vi "left shift.vi"(11 "2048 2":dbl[][](array[numeric])) -> (3 "2048":dbl[][](array[numeric]))   [LabVIEW 2015]
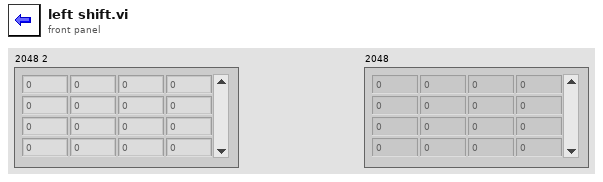
[diagram p1: front panel]
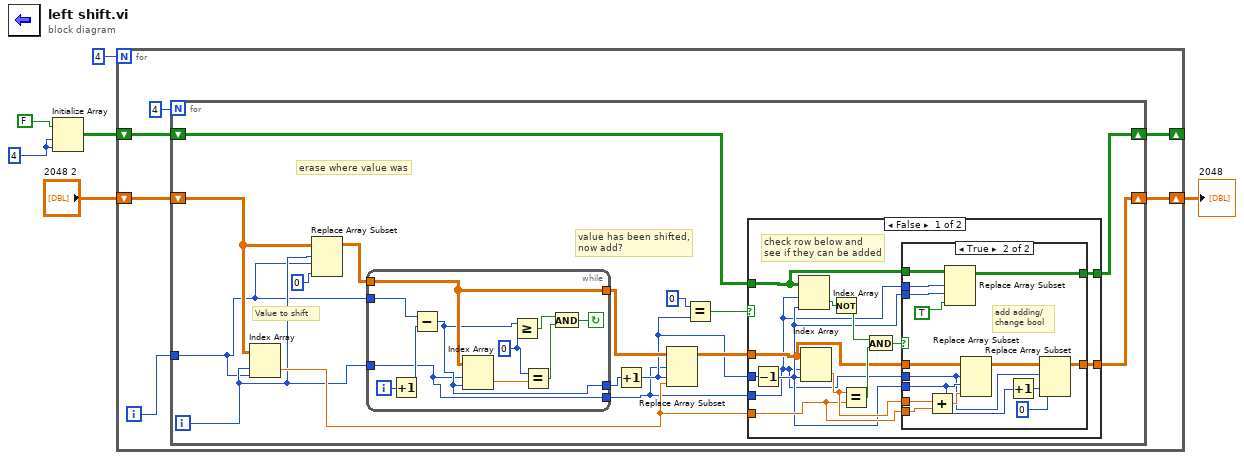
[diagram p0: block diagram]
diagram:
  w3 = 4
  n1 = Initialize Array(FALSE, w3, w3) -> (w1:bool[][])
  n2 = for {
    N: 4 -> [_]
    shift-right: [w8] -> _
    shift-left: w1 -> [w9]
    shift-right: [w7] -> w4
    shift-left: "2048 2" -> [w11]
    i -> [w10]
    n3 = for {
      N: 4 -> [_]
      tunnel: w10 -> [w13]
      shift-right: [w21] -> w8
      shift-left: w9 -> [w22]
      shift-right: [w20] -> w7
      shift-left: w11 -> [w18]
      i -> [w14]
      # "erase where value was"
      # "value has been shifted,\nnow add?"
      # "Value to shift"
      n4 = Index Array(array=w18, index (row)=w14, index (col)=w13) -> (element=w23:dbl)
      n5 = Replace Array Subset(array=w18, new element=0, index (row)=w14, index (col)=w13) -> (w19:dbl[][])
      n6 = while {
        tunnel: w13 -> [w71]
        tunnel: w14 -> [w62]
        tunnel: w19 -> [w64]
        tunnel: [w62] -> w15
        tunnel: [w63] -> w24
        tunnel: [w64] -> w28
        i -> [w70]
        stop <- w66 continue-if-true
        w61 = 0
        n7 = Increment(x=w70) -> (x+1=w67:i32)
        n8 = Subtract(x=w71, y=w67) -> (x-y=w63:i32)
        n9 = Index Array(array=w64, index (row)=w62, index (col)=w63) -> (element=w69:dbl)
        n10 = Greater Or Equal?(x=w63, y=w61) -> (x >= y?=w65:bool)
        n11 = Equal?(x=w61, y=w69) -> (x = y?=w68:bool)
        n12 = And(x=w65, y=w68) -> (x .and. y?=w66:bool)
      }
      n13 = Increment(x=w24) -> (x+1=w16:i32)
      n14 = Replace Array Subset(array=w28, new element=w23, index (row)=w15, index (col)=w16) -> (w25:dbl[][])
      n15 = Equal?(x=0, y=w16) -> (x = y?=w26:bool)
      n16 = case shown="False" w26 {
        tunnel: w25 -> [w35 w59]
        tunnel: w15 -> [w29 _]
        tunnel: w16 -> [w41 _]
        tunnel: w23 -> [w33 _]
        tunnel: w22 -> [w37 w60]
        tunnel: [w32 w60] -> w21
        tunnel: [w31 w59] -> w20
        frame False {
          # "check row below and \nsee if they can be added"
          n17 = Decrement(x=w41) -> (x-1=w30:i32)
          n18 = Index Array(array=w37, index (row)=w29, index (col)=w30) -> (element=w39:bool)
          n19 = Index Array(array=w35, index (row)=w29, index (col)=w30) -> (element=w34:dbl)
          n20 = Not(x=w39) -> (.not. x?=w38:bool)
          n21 = Equal?(x=w34, y=w33) -> (x = y?=w40:bool)
          n22 = And(x=w38, y=w40) -> (x .and. y?=w36:bool)
          n23 = case shown="True" w36 {
            tunnel: w37 -> [w43 w58]
            tunnel: w30 -> [_ w57]
            tunnel: w29 -> [_ w56]
            tunnel: w35 -> [w42 w54]
            tunnel: w29 -> [_ w44]
            tunnel: w30 -> [_ w46]
            tunnel: w34 -> [_ w52]
            tunnel: w33 -> [_ w51]
            tunnel: [w43 w50] -> w32
            tunnel: [w42 w48] -> w31
            frame False {
            }
            frame True {
              # "add adding/\nchange bool"
              n24 = Add(x=w52, y=w51) -> (x+y=w53:dbl)
              n25 = Replace Array Subset(array=w58, new element=TRUE, index (row)=w56, index (col)=w57) -> (w50:bool[][])
              n26 = Replace Array Subset(array=w54, new element=w53, index (row)=w44, index (col)=w46) -> (w49:dbl[][])
              n27 = Increment(x=w46) -> (x+1=w45:i32)
              n28 = Replace Array Subset(array=w49, new element=0, index (row)=w44, index (col)=w45) -> (w48:dbl[][])
            }
          }
        }
        frame True {
          # "if it is row 0 then,\n no adds to check"
        }
      }
    }
  }
  "2048" <- w4
